vi "for_T.vi"() -> ()   [LabVIEW 2019]
panel:
  out "x+y 3":u8
  out "x+y 2":u8
  out "x+y":u8
  out "x-y 3":u32
  out "x-y 2":u32
  out "x-y":u32
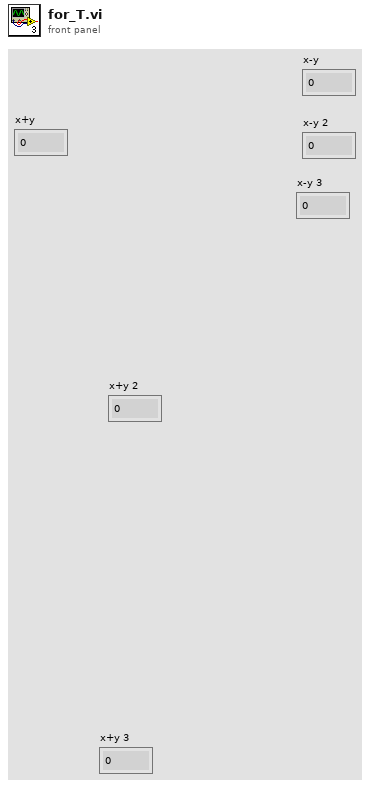
[diagram p1: front panel]
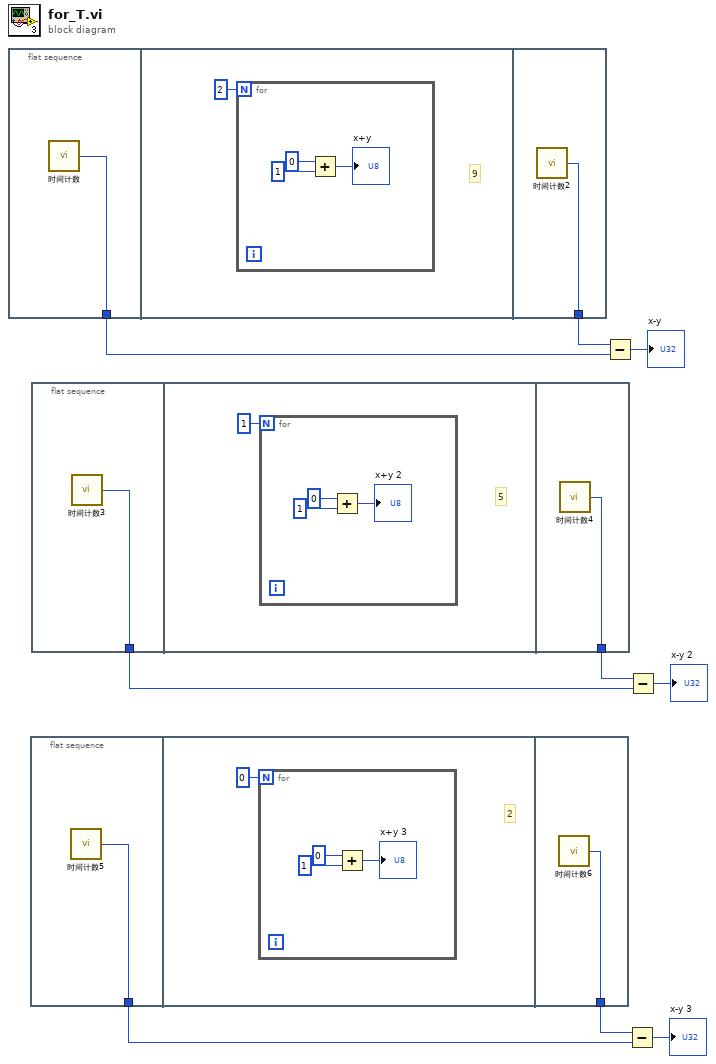
[diagram p0: block diagram]
diagram:
  n1 = flat-sequence {
    tunnel: [w10] -> w8
    tunnel: [w15] -> w9
    frame #0 {
      n2 = call "时间计数"() -> ("Tick Count(Ticks)"=w10:u32)
    }
    frame #1 {
      # "9"
      n3 = for {
        N: 2 -> [_]
        n4 = Add(x=u8 0, y=u8 1) -> (x+y=→"x+y":u8)
      }
    }
    frame #2 {
      n5 = call "时间计数2"() -> ("Tick Count(Ticks)"=w15:u32)
    }
  }
  n6 = flat-sequence {
    tunnel: [w16] -> w2
    tunnel: [w21] -> w3
    frame #0 {
      n7 = call "时间计数5"() -> ("Tick Count(Ticks)"=w16:u32)
    }
    frame #1 {
      # "2"
      n8 = for {
        N: 0 -> [_]
        n9 = Add(x=u8 0, y=u8 1) -> (x+y=→"x+y 3":u8)
      }
    }
    frame #2 {
      n10 = call "时间计数6"() -> ("Tick Count(Ticks)"=w21:u32)
    }
  }
  n11 = flat-sequence {
    tunnel: [w22] -> w5
    tunnel: [w27] -> w4
    frame #0 {
      n12 = call "时间计数3"() -> ("Tick Count(Ticks)"=w22:u32)
    }
    frame #1 {
      # "5"
      n13 = for {
        N: 1 -> [_]
        n14 = Add(x=u8 0, y=u8 1) -> (x+y=→"x+y 2":u8)
      }
    }
    frame #2 {
      n15 = call "时间计数4"() -> ("Tick Count(Ticks)"=w27:u32)
    }
  }
  n16 = Subtract(x=w9, y=w8) -> (x-y=→"x-y":u32)
  n17 = Subtract(x=w3, y=w2) -> (x-y=→"x-y 3":u32)
  n18 = Subtract(x=w4, y=w5) -> (x-y=→"x-y 2":u32)
